vi "BenchmarkLocalize.vi"() -> ()   [LabVIEW 2011]
uses:
  JelmersTracker.llb/TrackerDLL.vi
panel:
  in  "Image size":cluster{"width":u32, "height":u32}={"width"=150, "height"=150}
  in  "Show traces?":bool
  out "FPS":dbl
  out "Loop count":i32
  out "appended path":path
  in  "Show graphs":bool
  in  "Use debug library":bool
  in  "xcor_iterations":i32=2
  out "X profile":sgl[](graph)
  out "Y profile":sgl[](graph)
  out "Y result":sgl[](graph)
  out "True Y":dbl
  out "True X":dbl
  out "COM results":cluster{dbl, dbl}(graph)
  out "XCor results":cluster{dbl, dbl}(graph)
  in  "y center":dbl=75.0
  in  "x center":dbl=75.0 min=40.0 max=200.0
  out "X result":sgl[](graph)
  in  "spotsize":sgl=2.0 min=1 max=20
  in  "Stop loop":bool
  out "median":sgl
  out "xcorpos":cluster{"XCor X":sgl, "XCor Y":sgl}
  out "COM":cluster{"comX":sgl, "comY":sgl}
  out "Image":T1(plugin-control)
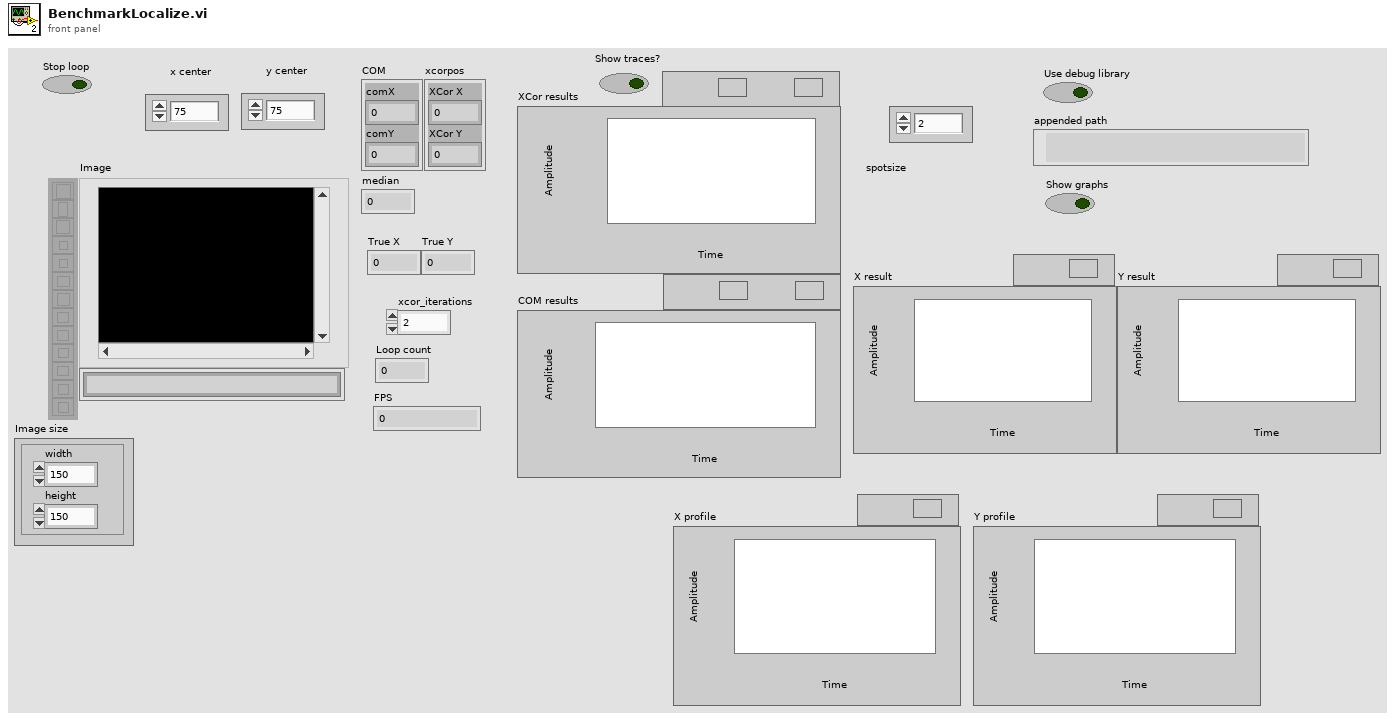
[diagram p1: front panel]
types:
  T1 = typedef "IMAQ Image.ctl" = refnum<image>
  T2 = typedef "Image Type" = u32
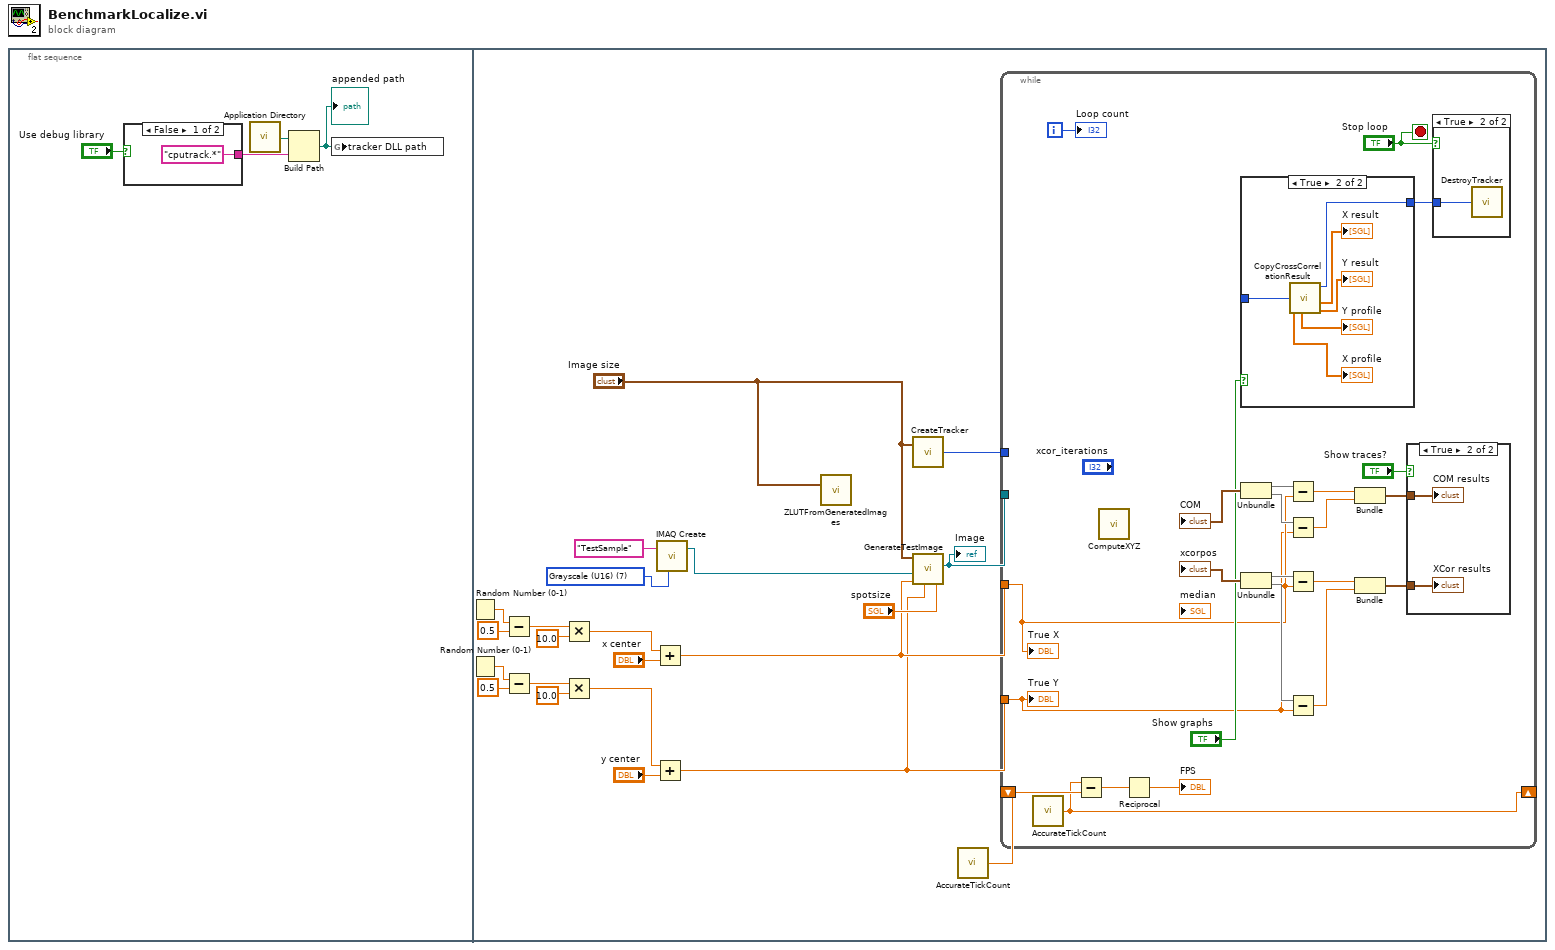
[diagram p0: block diagram]
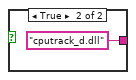
[diagram p2: hidden frame]
diagram:
  n1 = flat-sequence {
    frame #0 {
      n2 = case shown="False" "Use debug library" {
        tunnel: ["cputrack.*" "cputrack_d.dll"] -> w2
        frame False {
        }
        frame True {
        }
      }
      n3 = call <vilib>:"Application Directory.vi"() -> ("Application Directory"=w1:path)
      n4 = Build Path(base path=w1, name or relative path=w2) -> (appended path=w3:path)
      "appended path" <- w3
      n5 = global write "TrackerDLL.vi" "tracker DLL path"(w3) -> ()
    }
    frame #1 {
      w28 = T2 7 items=["Grayscale (U8)", "Grayscale (I16)", "Grayscale (SGL)", "Complex (CSG)", "RGB (U32)", "HSL (U32)", "RGB (U64)", "Grayscale (U16)"] ("Image Type")
      n6 = Random Number (0-1)() -> (number: 0 to 1=w18:dbl)
      n7 = Random Number (0-1)() -> (number: 0 to 1=w22:dbl)
      n8 = Subtract(x=w18, y=0.5) -> (x-y=w21:dbl)
      n9 = Subtract(x=w22, y=0.5) -> (x-y=w24:dbl)
      n10 = Multiply(x=w21, y=sgl 10.0) -> (x*y=w13:dbl)
      n11 = Multiply(x=w24, y=sgl 10.0) -> (x*y=w15:dbl)
      n12 = Add(x=w13, y="x center") -> (x+y=w11:dbl)
      n13 = Add(x=w15, y="y center") -> (x+y=w10:dbl)
      n14 = call "IMAQ Create"("Image Name"="TestSample" ("String"), "Image Type"=w28) -> ("New Image"=w9:T1)  [unwired: 3 in, 1 out]
      n15 = call "ZLUTFromGeneratedImages.vi"("Image size"="Image size") -> ()  [unwired: 11 in, 4 out]
      n16 = call "CreateTracker.vi"("Image size"="Image size") -> ("return type"=w26:u64)  [unwired: 1 in]
      n17 = call "GenerateTestImage.vi"("spotsize"="spotsize", "ypos"=w10, "xpos"=w11, "image"=w9, "Image size"="Image size") -> ("Image"=w8:T1)  [unwired: 4 in]
      "Image" <- w8
      n18 = call "AccurateTickCount.vi"() -> ("seconds"=w25:dbl)
      n19 = while {
        tunnel: w26 -> [w56]
        shift-right: [w36] -> _
        shift-left: w25 -> [w37]
        tunnel: w11 -> [w33]
        tunnel: w10 -> [w32]
        tunnel: w8 -> [w31]
        i -> [w38]
        stop <- "Stop loop" stop-if-true
        n20 = call "AccurateTickCount.vi"() -> ("seconds"=w36:dbl)
        n21 = Subtract(x=w36, y=w37) -> (x-y=w35:dbl)
        n22 = call "ComputeXYZ.vi"() -> ()  [unwired: 12 in]
        n23 = Reciprocal(x=w35) -> (1/x=→"FPS":dbl)
        n24 = case shown="True" "Show graphs" {
          tunnel: [w59 w65] -> w42
          tunnel: [w59 w64] -> w41
          frame False {
          }
          frame True {
            n25 = call "CopyCrossCorrelationResult.vi"("tracker"=w65) -> ("x prof"=→"X profile":sgl[], "y prof"=→"Y profile":sgl[], "tracker"=w64:u64, "x result"=→"X result":sgl[], "y_result"=→"Y result":sgl[])  [unwired: 3 in]
          }
        }
        n26 = Unbundle("COM") -> ("comX"=w44, "comY"=w43)
        n27 = Unbundle("xcorpos") -> ("XCor X"=w52, "XCor Y"=w51)
        n28 = Subtract(x=w44, y=w33) -> (x-y=w47:dbl)
        n29 = Subtract(x=w43, y=w32) -> (x-y=w46:dbl)
        n30 = Subtract(x=w52, y=w33) -> (x-y=w50:dbl)
        n31 = Subtract(x=w51, y=w32) -> (x-y=w49:dbl)
        n32 = Bundle(w47, w46) -> (w30:cluster{dbl, dbl})  [unwired: 1 in]
        n33 = Bundle(w50, w49) -> (w48:cluster{dbl, dbl})  [unwired: 1 in]
        n34 = case shown="True" "Show traces?" {
          tunnel: w48 -> [_ w58]
          tunnel: w30 -> [_ w57]
          frame False {
          }
          frame True {
            "XCor results" <- w58
            "COM results" <- w57
          }
        }
        n35 = case shown="True" "Stop loop" {
          tunnel: w41 -> [_ w66]
          frame False {
          }
          frame True {
            n36 = call "DestroyTracker.vi"("tracker"=w66) -> ()
          }
        }
        "True X" <- w33
        "True Y" <- w32
        "Loop count" <- w38
      }
    }
  }
